vi "Read Parameter Definition.vi"(8 "error in":errorcluster, 11 "parameter ref in":refnum<k20>) -> (0 "error out":errorcluster, 2 "parameter":T2, 3 "parameter ref out":refnum<k20>)   [LabVIEW 2020, in "AIM MIL-STD 1553 Import.lvlib"]
uses:
  AIM MIL-STD 1553 Import.lvlib
  Shared/Parameter Definition.ctl
  ec28d4f3-48db-496c-9f2c-9c0f463deb5e.vi
  Constants.vi
  6d544800-6714-4abe-8309-f249f0e90a5c.vi
  f79f91f8-0e14-439e-8c92-d2b7439f1fed.vi
  d88c7b1d-5fb1-494e-85d8-229d509e2db4.vi
  35fd3d51-91dd-4180-b9f7-7b084d6605af.vi
  505602a3-da8d-4664-8e75-0f9e10799a3b.vi
  6ee519c4-301c-4c84-a8cb-96ce99f5447e.vi
  be198a5b-80c8-4217-8a28-db41689b18fa.vi
  b2bdd28a-7ae2-470f-9b05-511610cb63d5.vi
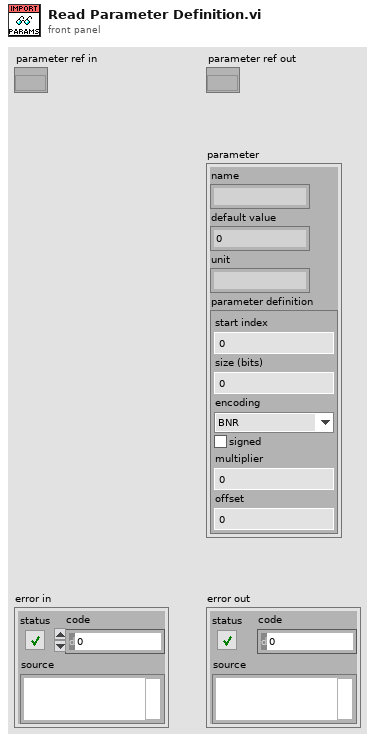
[diagram p1: front panel]
types:
  T1 = typedef "Parameter Definition.ctl" = cluster{"start index":i32, "size (bits)":i32, "encoding":enum16{"BNR", "BCD", "Discrete"}, "signed":bool, "multiplier":dbl, "offset":dbl}
  T2 = cluster{"name":string, "default value":dbl, "unit":string, "parameter definition":T1}
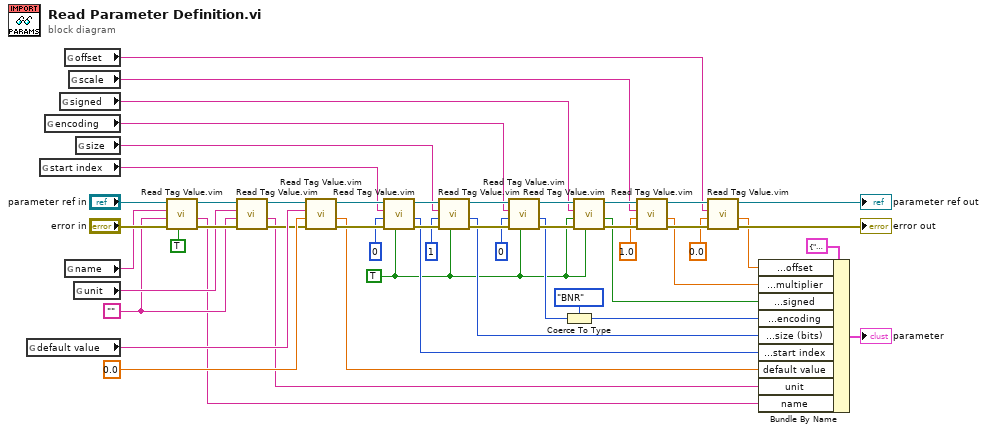
[diagram p0: block diagram]
diagram:
  w8 = TRUE ("required (F)")
  w38 = "" ("name")
  n1 = global read "Constants.vi" "default value"() -> (w47:string)
  n2 = global read "Constants.vi" "start index"() -> (w20:string)
  n3 = global read "Constants.vi" "encoding"() -> (w14:string)
  n4 = global read "Constants.vi" "signed"() -> (w9:string)
  n5 = global read "Constants.vi" "offset"() -> (w5:string)
  n6 = global read "Constants.vi" "name"() -> (w49:string)
  n7 = global read "Constants.vi" "scale"() -> (w6:string)
  n8 = global read "Constants.vi" "unit"() -> (w39:string)
  n9 = global read "Constants.vi" "size"() -> (w16:string)
  n10 = call "Read Tag Value.vim"("required (F)"=TRUE, "error in"="error in", "default"=w38, "tag name"=w49, "node in"="parameter ref in") -> ("error out"=w42:errorcluster, "value"=w26:string, "node out"=w43:refnum<k20>)  [unwired: 4 in]
  n11 = call "Read Tag Value.vim"("error in"=w42, "default"=w38, "tag name"=w39, "node in"=w43) -> ("error out"=w41:errorcluster, "value"=w22:string, "node out"=w40:refnum<k20>)  [unwired: 5 in]
  n12 = call "Read Tag Value.vim"("error in"=w41, "default"=0.0, "tag name"=w47, "node in"=w40) -> ("error out"=w44:errorcluster, "value"=w21:dbl, "node out"=w45:refnum<k20>)  [unwired: 5 in]
  n13 = call "Read Tag Value.vim"("required (F)"=w8, "error in"=w44, "default"=0, "tag name"=w20, "node in"=w45) -> ("error out"=w34:errorcluster, "value"=w18:i32, "node out"=w35:refnum<k20>)  [unwired: 4 in]
  n14 = call "Read Tag Value.vim"("required (F)"=w8, "error in"=w34, "default"=1, "tag name"=w16, "node in"=w35) -> ("error out"=w37:errorcluster, "value"=w15:i32, "node out"=w36:refnum<k20>)  [unwired: 4 in]
  n15 = call "Read Tag Value.vim"("required (F)"=w8, "error in"=w37, "default"=u16 0, "tag name"=w14, "node in"=w36) -> ("error out"=w28:errorcluster, "value"=w12:u16, "node out"=w29:refnum<k20>)  [unwired: 4 in]
  n16 = Coerce To Type(0:w12, 1:enum16{"BNR", "BCD", "Discrete"}."BNR" ("parameter definition.encoding")) -> (2:w10:enum16{"BNR", "BCD", "Discrete"})
  n17 = call "Read Tag Value.vim"("required (F)"=w8, "error in"=w28, "default"=w8, "tag name"=w9, "node in"=w29) -> ("error out"=w33:errorcluster, "value"=w7:bool, "node out"=w32:refnum<k20>)  [unwired: 4 in]
  n18 = call "Read Tag Value.vim"("error in"=w33, "default"=1.0, "tag name"=w6, "node in"=w32) -> ("error out"=w30:errorcluster, "value"=w2:dbl, "node out"=w31:refnum<k20>)  [unwired: 5 in]
  n19 = call "Read Tag Value.vim"("error in"=w30, "default"=0.0, "tag name"=w5, "node in"=w31) -> ("error out"=→"error out":errorcluster, "value"=w1:dbl, "node out"=→"parameter ref out":refnum<k20>)  [unwired: 5 in]
  n20 = Bundle By Name(cluster=T2 {"name"="", "default value"=1.0, "unit"="", "parameter definition"={"start index"=0, "size (bits)"=16, "encoding"=enum."BNR", "signed"=FALSE, "multiplier"=1.0, "offset"=0.0}} ("definition with default value"), "parameter definition.offset"=w1, "parameter definition.multiplier"=w2, "parameter definition.signed"=w7, "parameter definition.encoding"=w10, "parameter definition.size (bits)"=w15, "parameter definition.start index"=w18, "default value"=w21, "unit"=w22, "name"=w26) -> (→"parameter":T2)
